vi "zoom in range.vi"(6 "factor":i32=1, 11 "F Array in":dbl[](array[numeric])=[2732195.911317379, 2732215.911317379, 2732235.911317379, 2732255.911317379, 2732275.911317379, 2732295.911317379, 2732315.911317379, 2732335.911317379, 2732355.911317379, 2732375.911317379]) -> (0 "new min":dbl, 1 "new max":dbl, 2 "win":dbl, 3 "center":dbl)   [LabVIEW 2010]
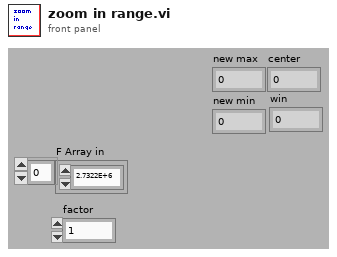
[diagram p1: front panel]
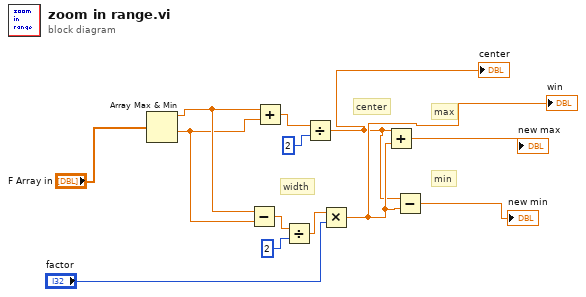
[diagram p0: block diagram]
diagram:
  # "min"
  # "max"
  # "width"
  # "center"
  n1 = Array Max & Min(array="F Array in") -> (max value=w10:dbl, min value=w9:dbl)  [unwired: 2 out]
  n2 = Subtract(x=w10, y=w9) -> (x-y=w6:dbl)
  n3 = Add(x=w10, y=w9) -> (x+y=w12:dbl)
  n4 = Divide(x=w6, y=2) -> (x/y=w5:dbl)
  n5 = Divide(x=w12, y=2) -> (x/y=w1:dbl)
  "center" <- w1
  n6 = Multiply(x=w5, y="factor") -> (x*y=w2:dbl)
  "win" <- w2
  n7 = Add(x=w1, y=w2) -> (x+y=→"new max":dbl)
  n8 = Subtract(x=w1, y=w2) -> (x-y=→"new min":dbl)
